vi "SMC_RangeMeasure.vi"(8 "error in (no error)":errorcluster) -> (0 "error out":errorcluster)   [LabVIEW 2015]
uses:
  SMC_SubVIs.llb/SMC_ManagerMode.ctl
  SMC_SubVIs.llb/glb_stop.vi
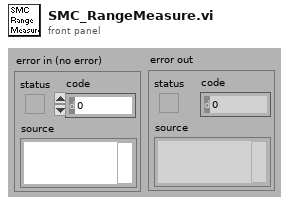
[diagram p1: front panel]
types:
  T1 = typedef "SMC_ManagerMode.ctl" = enum16{"Init", "Get", "SetPosition", "SetStatus", "SetMoving", "SetControllerNr"}
  T2 = typedef "SMC Paras.ctl" = cluster{"VENUS Language":T3, "Number of Axis":u8, "Controller Nr":u8, "Simulation":bool}
  T3 = typedef "VENUSNr.ctl" = enum16{"VENUS 2", "VENUS 1"}
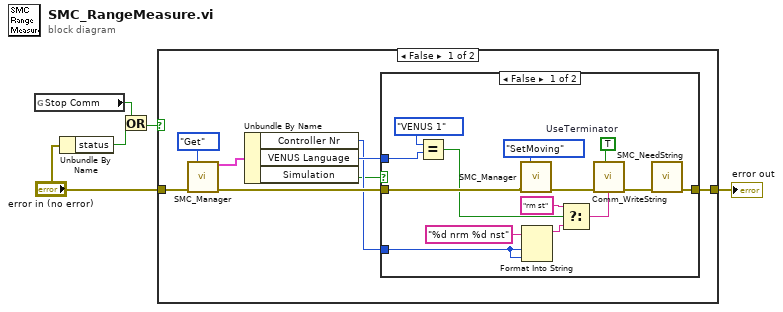
[diagram p0: block diagram]
diagram:
  n1 = global read "glb_stop.vi" "Stop Comm"() -> (w3:bool)
  n2 = Unbundle By Name("error in (no error)") -> ("status"=w1:bool)
  n3 = Or(x=w3, y=w1) -> (x .or. y?=w2:bool)
  n4 = case shown="False" w2 {
    tunnel: "error in (no error)" -> [w11 w29]
    tunnel: [w12 w29] -> w4
    frame False {
      n5 = call "SMC_Manager.vi"("Mode"=SMC_ManagerMode."Get", "error in (no error)"=w11) -> ("SMC Parameter Out"=w9:T2, "error out"=w10:errorcluster)  [unwired: 9 in, 3 out]
      n6 = Unbundle By Name(w9) -> ("Controller Nr"=w7:u8, "VENUS Language"=w8:T3, "Simulation"=w6:bool)
      n7 = case shown="False" w6 {
        tunnel: [w25 w28] -> w12
        tunnel: w10 -> [w24 w28]
        tunnel: w8 -> [w21 _]
        tunnel: w7 -> [w15 _]
        frame False {
          w14 = TRUE  # UseTerminator
          n8 = Equal?(x=enum16{"VENUS 2", "VENUS 1"}."VENUS 1", y=w21) -> (x = y?=w16:bool)
          n9 = call "SMC_Manager.vi"("Mode"=SMC_ManagerMode."SetMoving", "error in (no error)"=w24) -> ("error out"=w23:errorcluster)  [unwired: 9 in, 4 out]
          n10 = Format Into String(format string="%d nrm %d nst" ("Format String"), w15, w15) -> (resulting string=w19:string)  [unwired: 2 in, 1 out]
          n11 = Select(t="rm st" ("Substring"), s=w16, f=w19) -> (s? t:f=w17:string)
          n12 = call "Comm_WriteString.vi"("string to write"=w17, "error in (no error)"=w23, "UseTerminator"=w14) -> ("error out"=w26:errorcluster)  [unwired: 8 in]
          n13 = call "SMC_NeedString.vi"("error in (no error)"=w26) -> ("error out"=w25:errorcluster)  [unwired: 9 in, 1 out]
        }
        frame True {
          # "Simulation"
        }
      }
    }
    frame True {
      # "Error, do nothing"
    }
  }
  "error out" <- w4
